vi "Ground Griddy Manipulator Controls.vi"(8 "Stored Game Piece":T1=enum."Cone", 9 "Deadband":dbl=0.2 format="%#_13g", 10 "Driver Buttons":bool[](array[boolean]), 11 "Driver Axes":dbl[](array[numeric])) -> (3 "Ground Griddy Manipulator Controls":T2)   [LabVIEW 2020]
uses:
  manipulator/Implementation/Typedefs/Teleop Manipulator Commands.ctl
  manipulator/Implementation/Typedefs/game object.ctl
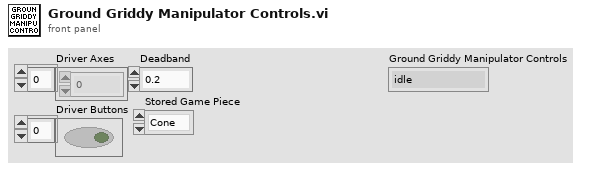
[diagram p1: front panel]
types:
  T1 = typedef "game object.ctl" = enum16{"Nothing", "Cone", "Cube"}
  T2 = typedef "Teleop Manipulator Commands.ctl" = enum16{"idle", "intake cone sideways", "intake cone upright", "intake cone feeder", "intake cube feeder", "intake cube", "score low cone", "score low cube", "score mid cone", "score mid cube", "score high cone", "score high cube", "score mid cone up"}
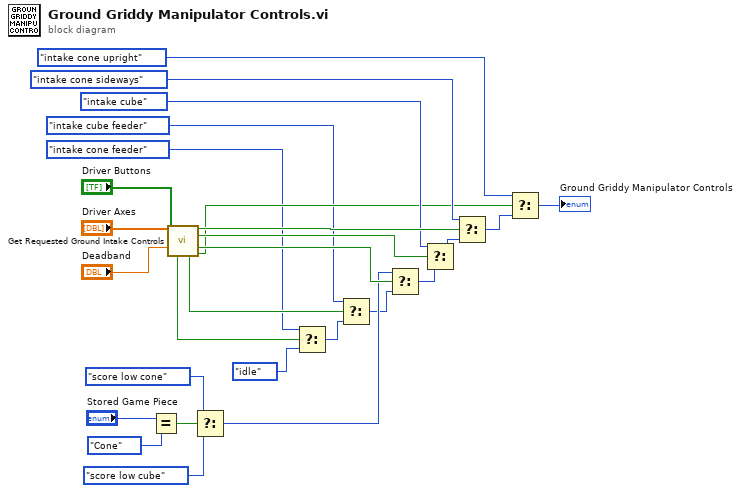
[diagram p0: block diagram]
diagram:
  n1 = Equal?(x="Stored Game Piece", y=game_object."Cone") -> (x = y?=w13:bool)
  n2 = call "Get Requested Ground Intake Controls.vi"("Driver Axes"="Driver Axes", "Driver Buttons"="Driver Buttons", "Deadband"="Deadband") -> ("Intake Sideways Cone Requested?"=w22:bool, "Intake Cube Requested?"=w21:bool, "Outtake Requested?"=w20:bool, "Intake Cone Feeder"=w4:bool, "Intake Cube Feeder"=w8:bool, "Intake Upright Cone Requested?"=w10:bool)  [unwired: 6 in, 1 out]
  n3 = Select(t=Teleop_Manipulator_Commands."score low cone" ("Griddy Command"), s=w13, f=Teleop_Manipulator_Commands."score low cube" ("Griddy Command")) -> (s? t:f=w17:T2)
  n4 = Select(t=Teleop_Manipulator_Commands."intake cone feeder" ("Griddy Command"), s=w4, f=Teleop_Manipulator_Commands."idle") -> (s? t:f=w2:T2)
  n5 = Select(t=Teleop_Manipulator_Commands."intake cube feeder" ("Griddy Command"), s=w8, f=w2) -> (s? t:f=w6:T2)
  n6 = Select(t=w17, s=w20, f=w6) -> (s? t:f=w23:T2)
  n7 = Select(t=Teleop_Manipulator_Commands."intake cube" ("Griddy Command"), s=w21, f=w23) -> (s? t:f=w24:T2)
  n8 = Select(t=Teleop_Manipulator_Commands."intake cone sideways" ("Griddy Command"), s=w22, f=w24) -> (s? t:f=w12:T2)
  n9 = Select(t=Teleop_Manipulator_Commands."intake cone upright", s=w10, f=w12) -> (s? t:f=→"Ground Griddy Manipulator Controls":T2)
